vi "LVUSBRH2_VISA_CMD_ver_Q.vi"(8 "error in (no error)":errorcluster caption="error in(no errro)", 11 "VISA rssc":refnum<visa-resource-name>) -> (0 "error out":errorcluster, 1 "recv string":string, 3 "VISA rssc out":refnum<visa-resource-name>)   [LabVIEW 2020]
panel:
  out "cmd string":string
  # "Response: \"uusbrh2, ver 1.0.0\""
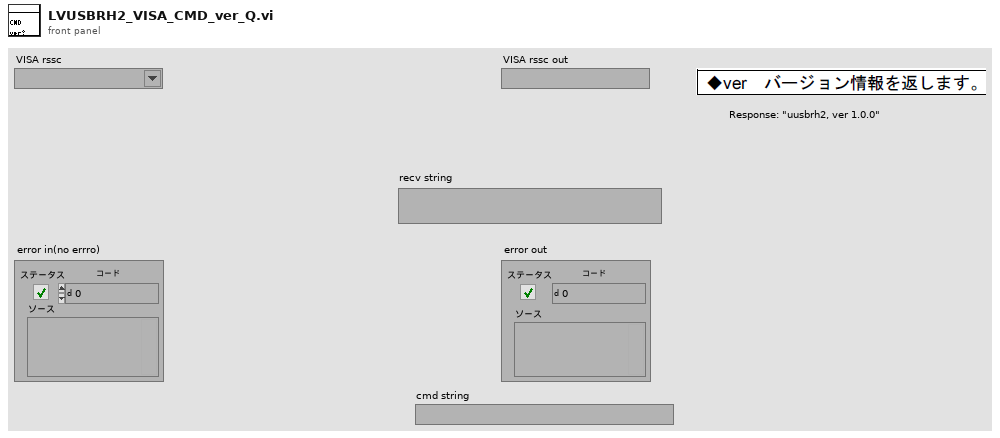
[diagram p1: front panel]
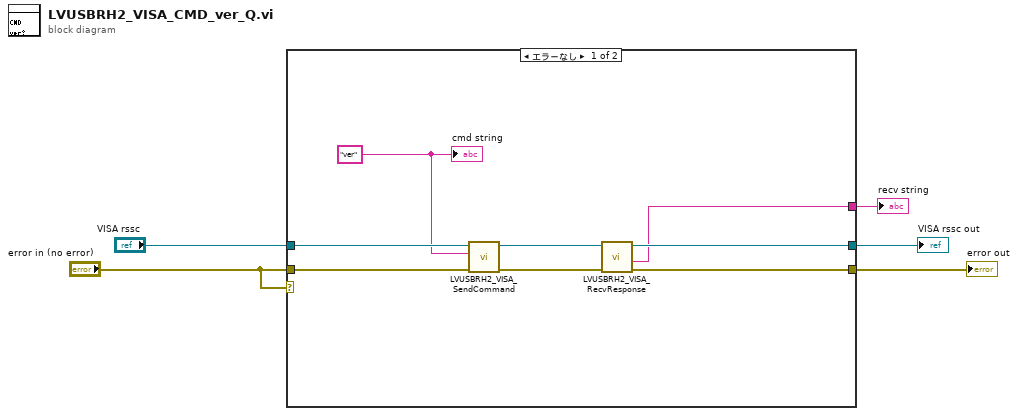
[diagram p0: block diagram]
diagram:
  n1 = case shown="エラーなし" "error in (no error)" {
    tunnel: "VISA rssc" -> [w13 w15]
    tunnel: [w10 w15] -> w4
    tunnel: "error in (no error)" -> [w12 w14]
    tunnel: [w7 w14] -> w3
    tunnel: [w6 _] -> w1
    frame No Error {
      w9 = "ver" ("形式文字列")
      n2 = call "LVUSBRH2_VISA_SendCommand.vi"("error in (no error)"=w12, "cmd string"=w9, "VISA rssc"=w13) -> ("error out"=w8:errorcluster, "VISA rssc out"=w11:refnum<visa-resource-name>)  [unwired: 7 in]
      n3 = call "LVUSBRH2_VISA_RecvResponse.vi"("error in (no error)"=w8, "VISA rssc"=w11) -> ("error out"=w7:errorcluster, "rcv string"=w6:string, "VISA rssc out"=w10:refnum<visa-resource-name>)  [unwired: 7 in]
      "cmd string" <- w9
    }
    frame Error {
    }
  }
  "VISA rssc out" <- w4
  "error out" <- w3
  "recv string" <- w1
